vi "HP34401_display_value.vi"(8 "error in":errorcluster, 9 "status code":i32, 10 "temp [deg C]":dbl, 11 "VISA in":refnum<visa-resource-name>) -> (0 "error out":errorcluster, 3 "VISA out":refnum<visa-resource-name>)   [LabVIEW 2020]
uses:
  drivers/HP34401A/Agilent 34401.lvlib
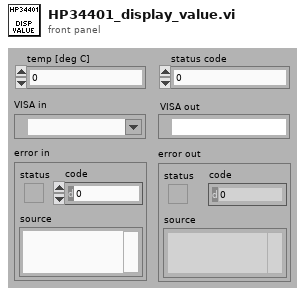
[diagram p1: front panel]
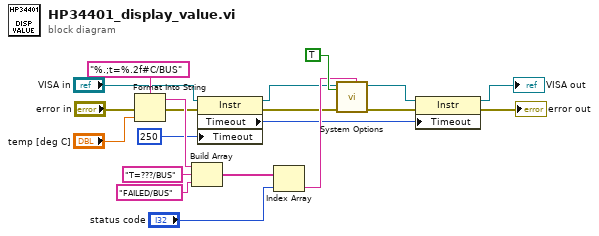
[diagram p0: block diagram]
diagram:
  n1 = Format Into String(format string="%.;t=%.2f#C/BUS", error in="error in", "temp [deg C]") -> (resulting string=w14:string, error out=w11:errorcluster)  [unwired: 1 in]
  n2 = Build Array(w14, "T=???/BUS" ("element"), "FAILED/BUS" ("element")) -> (w17:string[])
  n3 = property class="Instr"(reference="VISA in", error in=w11, "Timeout"=u32 250 ("General Settings:Timeout Value")) -> (reference out=w9:refnum<visa-resource-name>, error out=w3:errorcluster, "Timeout"=w4:u32)
  n4 = Index Array(array=w17, index="status code") -> (element=w16:string)
  n5 = call "System Options.vi"("Message Text (Empty)"=w16, "Message (F: OFF)"=TRUE, "error in (no error)"=w3, "VISA resource name"=w9) -> ("error out"=w8:errorcluster, "VISA resource name out"=w6:refnum<visa-resource-name>)  [unwired: 6 in]
  n6 = property class="Instr"(reference=w6, error in=w8, "Timeout"=w4) -> (reference out=→"VISA out":refnum<visa-resource-name>, error out=→"error out":errorcluster)
